vi "Read parametersFileRefnum.vi"(11 "Log in":refnum<class "Log.lvclass">) -> (2 "parametersFileRefnum":refnum<file>, 3 "Log out":refnum<class "Log.lvclass">)   [LabVIEW 2013, in "Log.lvlib" / "Log.lvclass"]
uses:
  <userlib>/Common/Log/Log/Log.lvclass
  <userlib>/Common/Log/Log/Log.lvclass/Log.ctl
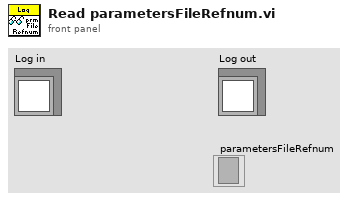
[diagram p1: front panel]
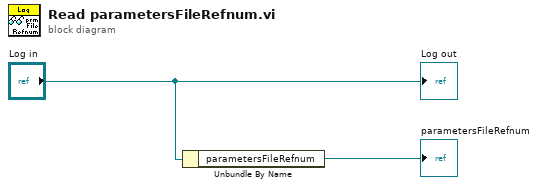
[diagram p0: block diagram]
diagram:
  n1 = Unbundle By Name("Log in") -> ("parametersFileRefnum"=→"parametersFileRefnum":refnum<file>)
  "Log out" <- "Log in"
